vi "Forward.vi"(1 "Speed":dbl, 2 "Driving Distance":dbl) -> ()   [LabVIEW 2018]
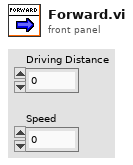
[diagram p1: front panel]
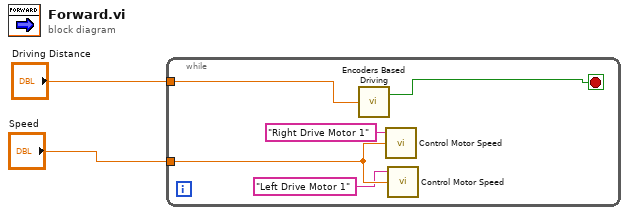
[diagram p0: block diagram]
diagram:
  n1 = while {
    tunnel: "Driving Distance" -> [w7]
    tunnel: "Speed" -> [w5]
    stop <- w6 stop-if-true
    n2 = call "Encoders Based Driving.vi"("Distance"=w7) -> ("Encoder Bigger Than Distance"=w6:bool)  [unwired: 1 out]
    n3 = call "Control Motor Speed.vi"("Speed"=w5, "Motor Name"="Right Drive Motor 1") -> ()  [unwired: 2 in]
    n4 = call "Control Motor Speed.vi"("Speed"=w5, "Motor Name"="Left Drive Motor 1") -> ()  [unwired: 2 in]
  }
